vi "VI Tree.vi"   [LabVIEW 2020, in "Yokogawa GX Series.lvlib"]
doc: "This is the instrument driver for the Yokogawa DX series Paperless Recorder. The VI Tree displays all the user-callable VIs of the instrument driver in an organized table."
uses:
  <instrlib>/Yokogawa GX Series/Yokogawa GX Series.lvlib
  <instrlib>/Yokogawa GX Series/Public/Data/Read Measurement Data (Analog 1Chan).vi
panel:
  # "(c) 2013-2018 Yokogawa Electric Corporation.  ALL RIGHTS RESERVED."
  # "SEE DIAGRAM\nFOR VI TREE."
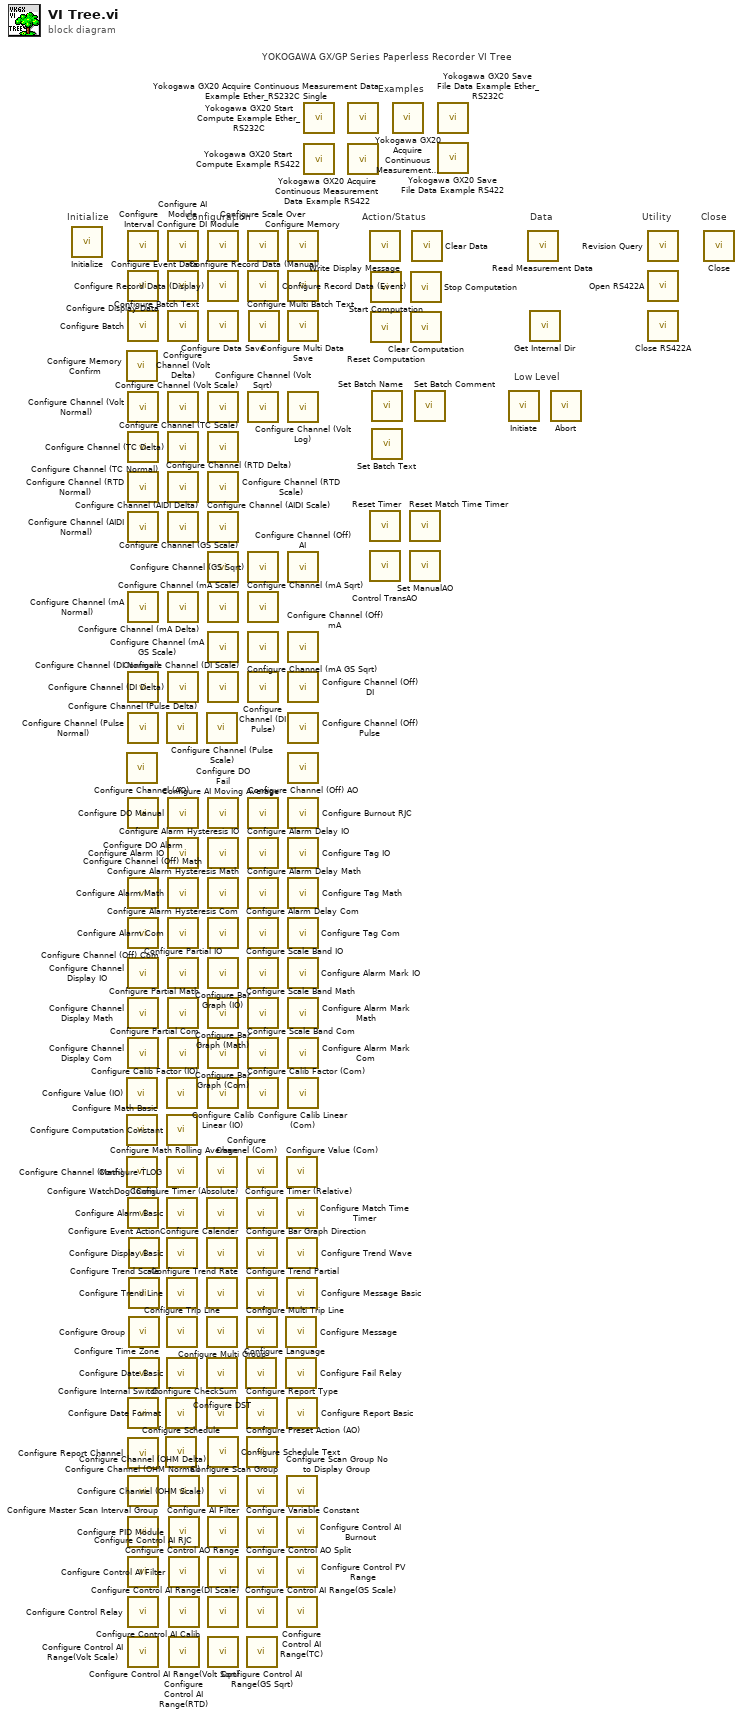
[diagram p0: block diagram]
diagram:
  # "YOKOGAWA GX/GP Series Paperless Recorder VI Tree"
  # "Examples"
  # "Low Level"
  # "Action/Status"
  # "Configuration"
  # "Utility"
  # "Data"
  # "Close"
  # "Initialize"
  n1 = call <instrlib>:"Initialize.vi"() -> ()  [unwired: 14 in, 2 out]
  n2 = call <instrlib>:"Configure Memory Confirm.vi"() -> ()  [unwired: 14 in, 2 out]
  n3 = call <instrlib>:"Configure Channel (AO).vi"() -> ()  [unwired: 25 in, 3 out]
  n4 = call <instrlib>:"Configure Value (IO).vi"() -> ()  [unwired: 13 in, 3 out]
  n5 = call <instrlib>:"Configure Math Basic.vi"() -> ()  [unwired: 14 in, 2 out]
  n6 = call <instrlib>:"Configure Channel (Math).vi"() -> ()  [unwired: 13 in, 3 out]
  n7 = call <instrlib>:"Configure Interval.vi"() -> ()  [unwired: 13 in, 3 out]
  n8 = call <instrlib>:"Configure Display Data.vi"() -> ()  [unwired: 14 in, 2 out]
  n9 = call <instrlib>:"Configure Batch.vi"() -> ()  [unwired: 14 in, 2 out]
  n10 = call <instrlib>:"Configure Channel (Volt Normal).vi"() -> ()  [unwired: 13 in, 3 out]
  n11 = call <instrlib>:"Configure Channel (TC Normal).vi"() -> ()  [unwired: 13 in, 3 out]
  n12 = call <instrlib>:"Configure Channel (RTD Normal).vi"() -> ()  [unwired: 13 in, 3 out]
  n13 = call <instrlib>:"Configure Channel (AIDI Normal).vi"() -> ()  [unwired: 13 in, 3 out]
  n14 = call <instrlib>:"Configure Channel (mA Normal).vi"() -> ()  [unwired: 13 in, 3 out]
  n15 = call <instrlib>:"Configure Channel (DI Normal).vi"() -> ()  [unwired: 13 in, 3 out]
  n16 = call <instrlib>:"Configure Channel (Pulse Normal).vi"() -> ()  [unwired: 25 in, 3 out]
  n17 = call <instrlib>:"Configure DO Alarm.vi"() -> ()  [unwired: 13 in, 3 out]
  n18 = call <instrlib>:"Configure Channel (Off) Math.vi"() -> ()  [unwired: 13 in, 3 out]
  n19 = call <instrlib>:"Configure Channel (Off) Com.vi"() -> ()  [unwired: 13 in, 3 out]
  n20 = call <instrlib>:"Configure Channel Display IO.vi"() -> ()  [unwired: 13 in, 3 out]
  n21 = call <instrlib>:"Configure Channel Display Math.vi"() -> ()  [unwired: 13 in, 3 out]
  n22 = call <instrlib>:"Configure Channel Display Com.vi"() -> ()  [unwired: 13 in, 3 out]
  n23 = call <instrlib>:"Configure WatchDog (Com).vi"() -> ()  [unwired: 13 in, 3 out]
  n24 = call <instrlib>:"Configure Internal Switch.vi"() -> ()  [unwired: 13 in, 3 out]
  n25 = call <instrlib>:"Configure Report Channel.vi"() -> ()  [unwired: 14 in, 2 out]
  n26 = call <instrlib>:"Configure Channel (OHM Delta).vi"() -> ()  [unwired: 13 in, 3 out]
  n27 = call <instrlib>:"Configure Master Scan Interval Group.vi"() -> ()  [unwired: 14 in, 2 out]
  n28 = call <instrlib>:"Configure Control AI RJC.vi"() -> ()  [unwired: 23 in, 5 out]
  n29 = call <instrlib>:"Configure Control Relay.vi"() -> ()  [unwired: 23 in, 5 out]
  n30 = call <instrlib>:"Configure Control AI Range(Volt Scale).vi"() -> ()  [unwired: 23 in, 5 out]
  n31 = call <instrlib>:"Configure Event Action.vi"() -> ()  [unwired: 13 in, 3 out]
  n32 = call <instrlib>:"Configure Trend Scale.vi"() -> ()  [unwired: 14 in, 2 out]
  n33 = call <instrlib>:"Configure Group.vi"() -> ()  [unwired: 13 in, 3 out]
  n34 = call <instrlib>:"Configure Time Zone.vi"() -> ()  [unwired: 14 in, 2 out]
  n35 = call <instrlib>:"Configure Date Format.vi"() -> ()  [unwired: 14 in, 2 out]
  n36 = call <instrlib>:"Configure Schedule.vi"() -> ()  [unwired: 26 in, 2 out]
  n37 = call <instrlib>:"Configure Channel (Pulse Delta).vi"() -> ()  [unwired: 17 in, 3 out]
  n38 = call <instrlib>:"Configure Calib Factor (IO).vi"() -> ()  [unwired: 13 in, 3 out]
  n39 = call <instrlib>:"Configure Computation Constant.vi"() -> ()  [unwired: 13 in, 3 out]
  n40 = call <instrlib>:"Configure TLOG.vi"() -> ()  [unwired: 13 in, 3 out]
  n41 = call <instrlib>:"Configure Alarm Basic.vi"() -> ()  [unwired: 14 in, 2 out]
  n42 = call <instrlib>:"Configure Display Basic.vi"() -> ()  [unwired: 14 in, 2 out]
  n43 = call <instrlib>:"Configure Trend Line.vi"() -> ()  [unwired: 14 in, 2 out]
  n44 = call <instrlib>:"Configure Trip Line.vi"() -> ()  [unwired: 12 in, 4 out]
  n45 = call <instrlib>:"Configure Date Basic.vi"() -> ()  [unwired: 14 in, 2 out]
  n46 = call <instrlib>:"Configure AI Module.vi"() -> ()  [unwired: 12 in, 4 out]
  n47 = call <instrlib>:"Configure Event Data.vi"() -> ()  [unwired: 13 in, 3 out]
  n48 = call <instrlib>:"Configure Batch Text.vi"() -> ()  [unwired: 13 in, 3 out]
  n49 = call <instrlib>:"Configure Channel (Volt Delta).vi"() -> ()  [unwired: 13 in, 3 out]
  n50 = call <instrlib>:"Configure Channel (TC Delta).vi"() -> ()  [unwired: 13 in, 3 out]
  n51 = call <instrlib>:"Configure Channel (RTD Delta).vi"() -> ()  [unwired: 13 in, 3 out]
  n52 = call <instrlib>:"Configure Channel (AIDI Delta).vi"() -> ()  [unwired: 13 in, 3 out]
  n53 = call <instrlib>:"Configure Channel (mA Delta).vi"() -> ()  [unwired: 13 in, 3 out]
  n54 = call <instrlib>:"Configure Channel (DI Delta).vi"() -> ()  [unwired: 13 in, 3 out]
  n55 = call <instrlib>:"Configure DO Manual.vi"() -> ()  [unwired: 13 in, 3 out]
  n56 = call <instrlib>:"Configure Alarm IO.vi"() -> ()  [unwired: 12 in, 4 out]
  n57 = call <instrlib>:"Configure Alarm Math.vi"() -> ()  [unwired: 12 in, 4 out]
  n58 = call <instrlib>:"Configure Alarm Com.vi"() -> ()  [unwired: 12 in, 4 out]
  n59 = call <instrlib>:"Configure Partial IO.vi"() -> ()  [unwired: 13 in, 3 out]
  n60 = call <instrlib>:"Configure Partial Math.vi"() -> ()  [unwired: 13 in, 3 out]
  n61 = call <instrlib>:"Configure Partial Com.vi"() -> ()  [unwired: 13 in, 3 out]
  n62 = call <instrlib>:"Configure Channel (OHM Normal).vi"() -> ()  [unwired: 13 in, 3 out]
  n63 = call <instrlib>:"Configure PID Module.vi"() -> ()  [unwired: 12 in, 4 out]
  n64 = call <instrlib>:"Configure Control AI Filter.vi"() -> ()  [unwired: 11 in, 5 out]
  n65 = call <instrlib>:"Configure Control AI Calib.vi"() -> ()  [unwired: 11 in, 5 out]
  n66 = call <instrlib>:"Configure Control AI Range(RTD).vi"() -> ()  [unwired: 23 in, 5 out]
  n67 = call <instrlib>:"Configure Channel (Pulse Scale).vi"() -> ()  [unwired: 17 in, 3 out]
  n68 = call <instrlib>:"Configure Math Rolling Average.vi"() -> ()  [unwired: 13 in, 3 out]
  n69 = call <instrlib>:"Configure Timer (Absolute).vi"() -> ()  [unwired: 13 in, 3 out]
  n70 = call <instrlib>:"Configure Calender.vi"() -> ()  [unwired: 14 in, 2 out]
  n71 = call <instrlib>:"Configure Trend Rate.vi"() -> ()  [unwired: 14 in, 2 out]
  n72 = call <instrlib>:"Configure Multi Group.vi"() -> ()  [unwired: 16 in, 4 out]
  n73 = call <instrlib>:"Configure DST.vi"() -> ()  [unwired: 14 in, 2 out]
  n74 = call <instrlib>:"Configure CheckSum.vi"() -> ()  [unwired: 14 in, 2 out]
  n75 = call <instrlib>:"Configure DI Module.vi"() -> ()  [unwired: 12 in, 4 out]
  n76 = call <instrlib>:"Configure Record Data (Display).vi"() -> ()  [unwired: 13 in, 3 out]
  n77 = call <instrlib>:"Configure Data Save.vi"() -> ()  [unwired: 14 in, 2 out]
  n78 = call <instrlib>:"Configure Channel (Volt Scale).vi"() -> ()  [unwired: 13 in, 3 out]
  n79 = call <instrlib>:"Configure Channel (TC Scale).vi"() -> ()  [unwired: 13 in, 3 out]
  n80 = call <instrlib>:"Configure Channel (RTD Scale).vi"() -> ()  [unwired: 13 in, 3 out]
  n81 = call <instrlib>:"Configure Channel (AIDI Scale).vi"() -> ()  [unwired: 13 in, 3 out]
  n82 = call <instrlib>:"Configure Channel (GS Scale).vi"() -> ()  [unwired: 13 in, 3 out]
  n83 = call <instrlib>:"Configure Channel (mA Scale).vi"() -> ()  [unwired: 13 in, 3 out]
  n84 = call <instrlib>:"Configure Channel (mA GS Scale).vi"() -> ()  [unwired: 13 in, 3 out]
  n85 = call <instrlib>:"Configure Channel (DI Scale).vi"() -> ()  [unwired: 13 in, 3 out]
  n86 = call <instrlib>:"Configure DO Fail.vi"() -> ()  [unwired: 13 in, 3 out]
  n87 = call <instrlib>:"Configure Alarm Hysteresis IO.vi"() -> ()  [unwired: 12 in, 4 out]
  n88 = call <instrlib>:"Configure Alarm Hysteresis Math.vi"() -> ()  [unwired: 12 in, 4 out]
  n89 = call <instrlib>:"Configure Alarm Hysteresis Com.vi"() -> ()  [unwired: 12 in, 4 out]
  n90 = call <instrlib>:"Configure Bar Graph (IO).vi"() -> ()  [unwired: 13 in, 3 out]
  n91 = call <instrlib>:"Configure Bar Graph (Math).vi"() -> ()  [unwired: 13 in, 3 out]
  n92 = call <instrlib>:"Configure Bar Graph (Com).vi"() -> ()  [unwired: 13 in, 3 out]
  n93 = call <instrlib>:"Configure Calib Linear (IO).vi"() -> ()  [unwired: 13 in, 3 out]
  n94 = call <instrlib>:"Configure Schedule Text.vi"() -> ()  [unwired: 18 in, 2 out]
  n95 = call <instrlib>:"Configure Channel (OHM Scale).vi"() -> ()  [unwired: 13 in, 3 out]
  n96 = call <instrlib>:"Configure AI Filter.vi"() -> ()  [unwired: 13 in, 3 out]
  n97 = call <instrlib>:"Configure Control AO Range.vi"() -> ()  [unwired: 11 in, 5 out]
  n98 = call <instrlib>:"Configure Control AI Range(DI Scale).vi"() -> ()  [unwired: 23 in, 5 out]
  n99 = call <instrlib>:"Configure Control AI Range(Volt Sqrt).vi"() -> ()  [unwired: 23 in, 5 out]
  n100 = call <instrlib>:"Configure Language.vi"() -> ()  [unwired: 14 in, 2 out]
  n101 = call <instrlib>:"Configure Channel (Com).vi"() -> ()  [unwired: 13 in, 3 out]
  n102 = call <instrlib>:"Configure Timer (Relative).vi"() -> ()  [unwired: 13 in, 3 out]
  n103 = call <instrlib>:"Configure Bar Graph Direction.vi"() -> ()  [unwired: 14 in, 2 out]
  n104 = call <instrlib>:"Configure Trend Partial.vi"() -> ()  [unwired: 14 in, 2 out]
  n105 = call <instrlib>:"Configure Multi Trip Line.vi"() -> ()  [unwired: 23 in, 5 out]
  n106 = call <instrlib>:"Configure Report Type.vi"() -> ()  [unwired: 14 in, 2 out]
  n107 = call <instrlib>:"Configure Preset Action (AO).vi"() -> ()  [unwired: 18 in, 2 out]
  n108 = call <instrlib>:"Configure Scan Group.vi"() -> ()  [unwired: 12 in, 4 out]
  n109 = call <instrlib>:"Configure Variable Constant.vi"() -> ()  [unwired: 13 in, 3 out]
  n110 = call <instrlib>:"Configure Control AO Split.vi"() -> ()  [unwired: 11 in, 5 out]
  n111 = call <instrlib>:"Configure Control AI Range(GS Scale).vi"() -> ()  [unwired: 23 in, 5 out]
  n112 = call <instrlib>:"Configure Control AI Range(GS Sqrt).vi"() -> ()  [unwired: 23 in, 5 out]
  n113 = call <instrlib>:"Configure Scale Over.vi"() -> ()  [unwired: 14 in, 2 out]
  n114 = call <instrlib>:"Configure Record Data (Event).vi"() -> ()  [unwired: 13 in, 3 out]
  n115 = call <instrlib>:"Configure Channel (Volt Sqrt).vi"() -> ()  [unwired: 13 in, 3 out]
  n116 = call <instrlib>:"Configure Channel (GS Sqrt).vi"() -> ()  [unwired: 13 in, 3 out]
  n117 = call <instrlib>:"Configure Channel (mA Sqrt).vi"() -> ()  [unwired: 13 in, 3 out]
  n118 = call <instrlib>:"Configure Channel (mA GS Sqrt).vi"() -> ()  [unwired: 13 in, 3 out]
  n119 = call <instrlib>:"Configure Channel (DI Pulse).vi"() -> ()  [unwired: 13 in, 3 out]
  n120 = call <instrlib>:"Configure AI Moving Average.vi"() -> ()  [unwired: 13 in, 3 out]
  n121 = call <instrlib>:"Configure Alarm Delay IO.vi"() -> ()  [unwired: 13 in, 3 out]
  n122 = call <instrlib>:"Configure Alarm Delay Math.vi"() -> ()  [unwired: 13 in, 3 out]
  n123 = call <instrlib>:"Configure Alarm Delay Com.vi"() -> ()  [unwired: 13 in, 3 out]
  n124 = call <instrlib>:"Configure Scale Band IO.vi"() -> ()  [unwired: 13 in, 3 out]
  n125 = call <instrlib>:"Configure Scale Band Math.vi"() -> ()  [unwired: 13 in, 3 out]
  n126 = call <instrlib>:"Configure Scale Band Com.vi"() -> ()  [unwired: 13 in, 3 out]
  n127 = call <instrlib>:"Configure Calib Factor (Com).vi"() -> ()  [unwired: 13 in, 3 out]
  n128 = call <instrlib>:"Configure Multi Batch Text.vi"() -> ()  [unwired: 16 in, 4 out]
  n129 = call <instrlib>:"Configure Message.vi"() -> ()  [unwired: 13 in, 3 out]
  n130 = call <instrlib>:"Configure Fail Relay.vi"() -> ()  [unwired: 14 in, 2 out]
  n131 = call <instrlib>:"Configure Value (Com).vi"() -> ()  [unwired: 13 in, 3 out]
  n132 = call <instrlib>:"Configure Match Time Timer.vi"() -> ()  [unwired: 13 in, 3 out]
  n133 = call <instrlib>:"Configure Trend Wave.vi"() -> ()  [unwired: 14 in, 2 out]
  n134 = call <instrlib>:"Configure Message Basic.vi"() -> ()  [unwired: 16 in]
  n135 = call <instrlib>:"Configure Report Basic.vi"() -> ()  [unwired: 14 in, 2 out]
  n136 = call <instrlib>:"Configure Scan Group No to Display Group.vi"() -> ()  [unwired: 13 in, 3 out]
  n137 = call <instrlib>:"Configure Control AI Burnout.vi"() -> ()  [unwired: 11 in, 5 out]
  n138 = call <instrlib>:"Configure Control PV Range.vi"() -> ()  [unwired: 14 in, 2 out]
  n139 = call <instrlib>:"Configure Control AI Range(TC).vi"() -> ()  [unwired: 23 in, 5 out]
  n140 = call <instrlib>:"Configure Memory.vi"() -> ()  [unwired: 14 in, 2 out]
  n141 = call <instrlib>:"Configure Record Data (Manual).vi"() -> ()  [unwired: 13 in, 3 out]
  n142 = call <instrlib>:"Configure Multi Data Save.vi"() -> ()  [unwired: 18 in, 2 out]
  n143 = call <instrlib>:"Configure Channel (Volt Log).vi"() -> ()  [unwired: 13 in, 3 out]
  n144 = call <instrlib>:"Configure Channel (Off) AI.vi"() -> ()  [unwired: 13 in, 3 out]
  n145 = call <instrlib>:"Configure Channel (Off) mA.vi"() -> ()  [unwired: 13 in, 3 out]
  n146 = call <instrlib>:"Configure Channel (Off) DI.vi"() -> ()  [unwired: 13 in, 3 out]
  n147 = call <instrlib>:"Configure Channel (Off) Pulse.vi"() -> ()  [unwired: 9 in, 3 out]
  n148 = call <instrlib>:"Configure Channel (Off) AO.vi"() -> ()  [unwired: 9 in, 3 out]
  n149 = call <instrlib>:"Configure Burnout RJC.vi"() -> ()  [unwired: 13 in, 3 out]
  n150 = call <instrlib>:"Configure Tag IO.vi"() -> ()  [unwired: 13 in, 3 out]
  n151 = call <instrlib>:"Configure Tag Math.vi"() -> ()  [unwired: 13 in, 3 out]
  n152 = call <instrlib>:"Configure Tag Com.vi"() -> ()  [unwired: 13 in, 3 out]
  n153 = call <instrlib>:"Configure Alarm Mark IO.vi"() -> ()  [unwired: 13 in, 3 out]
  n154 = call <instrlib>:"Configure Alarm Mark Math.vi"() -> ()  [unwired: 13 in, 3 out]
  n155 = call <instrlib>:"Configure Alarm Mark Com.vi"() -> ()  [unwired: 13 in, 3 out]
  n156 = call <instrlib>:"Configure Calib Linear (Com).vi"() -> ()  [unwired: 13 in, 3 out]
  n157 = call <instrlib>:"Yokogawa GX20 Start Compute Example Ether_RS232C.vi"() -> ()  [unwired: 12 in]
  n158 = call <instrlib>:"Yokogawa GX20 Start Compute Example RS422.vi"() -> ()  [unwired: 12 in]
  n159 = call <instrlib>:"Yokogawa GX20 Acquire Continuous Measurement Data Example Ether_RS232C Single.vi"() -> ()  [unwired: 12 in]
  n160 = call <instrlib>:"Yokogawa GX20 Acquire Continuous Measurement Data Example RS422.vi"() -> ()  [unwired: 12 in]
  n161 = call <instrlib>:"Write Display Message.vi"() -> ()  [unwired: 14 in, 2 out]
  n162 = call <instrlib>:"Reset Timer.vi"() -> ()  [unwired: 10 in, 2 out]
  n163 = call <instrlib>:"Control TransAO.vi"() -> ()  [unwired: 14 in, 2 out]
  n164 = call <instrlib>:"Start Computation.vi"() -> ()  [unwired: 10 in, 2 out]
  n165 = call <instrlib>:"Reset Computation.vi"() -> ()  [unwired: 10 in, 2 out]
  n166 = call <instrlib>:"Set Batch Name.vi"() -> ()  [unwired: 14 in, 2 out]
  n167 = call <instrlib>:"Set Batch Text.vi"() -> ()  [unwired: 14 in, 2 out]
  n168 = call <instrlib>:"Yokogawa GX20 Acquire Continuous Measurement Data Example Ether Multiple.vi"() -> ()  [unwired: 12 in]
  n169 = call <instrlib>:"Reset Match Time Timer.vi"() -> ()  [unwired: 10 in, 2 out]
  n170 = call <instrlib>:"Set ManualAO.vi"() -> ()  [unwired: 9 in, 3 out]
  n171 = call <instrlib>:"Stop Computation.vi"() -> ()  [unwired: 10 in, 2 out]
  n172 = call <instrlib>:"Clear Computation.vi"() -> ()  [unwired: 10 in, 2 out]
  n173 = call <instrlib>:"Clear Data.vi"() -> ()  [unwired: 14 in, 2 out]
  n174 = call <instrlib>:"Set Batch Comment.vi"() -> ()  [unwired: 14 in, 2 out]
  n175 = call <instrlib>:"Yokogawa GX20 Save File Data Example Ether_RS232C.vi"() -> ()  [unwired: 12 in]
  n176 = call <instrlib>:"Yokogawa GX20 Save File Data Example RS422.vi"() -> ()  [unwired: 12 in]
  n177 = call <instrlib>:"Initiate.vi"() -> ()  [unwired: 10 in, 2 out]
  n178 = call-poly <instrlib>:"Read Measurement Data.vi"() -> ()  [unwired: 8 in, 8 out]
  n179 = call <instrlib>:"Get Internal Dir.vi"() -> ()  [unwired: 11 in, 5 out]
  n180 = call <instrlib>:"Abort.vi"() -> ()  [unwired: 10 in, 2 out]
  n181 = call <instrlib>:"Revision Query.vi"() -> ()  [unwired: 8 in, 4 out]
  n182 = call <instrlib>:"Open RS422A.vi"() -> ()  [unwired: 10 in, 2 out]
  n183 = call <instrlib>:"Close RS422A.vi"() -> ()  [unwired: 10 in, 2 out]
  n184 = call <instrlib>:"Close.vi"() -> ()  [unwired: 11 in, 1 out]
